vi "RSZVB Marker Bandfilter Results ZVR.vi"(8 "error in (no error)":errorcluster {"code" format="%.0x"}, 9 "Marker (1)":i32=1, 10 "Channel (Trace) (1)":i32=1, 11 "VISA session":refnum<visa-resource-name>) -> (0 "error out":errorcluster {"code" format="%.0x"}, 1 "Bandwidth":dbl format="%^.3e", 3 "dup VISA session":refnum<visa-resource-name>)   [LabVIEW 2011]
doc: "This VI returns the results of a bandpass or a bandstop filter search.\n\nNote(s):\n\n(1) This VI is ZVR compatible.\n\nRemote-control command(s):\nCALCulate<Ch/Tr>:MARKer<Mk>:FUNCtion:BWIDth?"
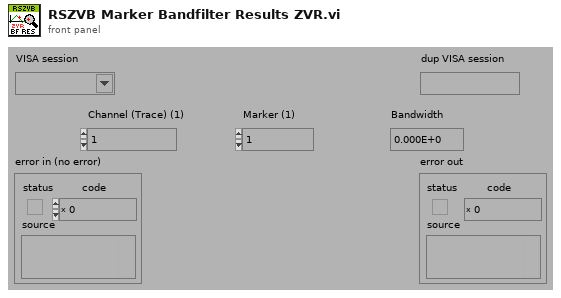
[diagram p1: front panel]
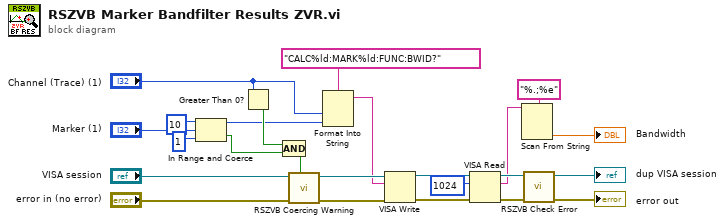
[diagram p0: block diagram]
diagram:
  n1 = In Range and Coerce(upper limit=10, x="Marker (1)", lower limit=1) -> (coerced(x)=w2:i32, In Range?=w12:bool)
  n2 = Greater Than 0?(x="Channel (Trace) (1)") -> (x > 0?=w15:bool)
  n3 = Compound Arithmetic op=AND(w15, w12) -> (w16:bool)
  n4 = call "RSZVB Coercing Warning.vi"("In Range?"=w16, "error in (no error)"="error in (no error)", "VISA session"="VISA session") -> ("error out"=w7:errorcluster, "dup VISA session"=w8:refnum<visa-resource-name>)  [unwired: 7 in]
  n5 = Format Into String(format string="CALC%ld:MARK%ld:FUNC:BWID?", "Channel (Trace) (1)", w2) -> (resulting string=w6:string)  [unwired: 2 in, 1 out]
  n6 = VISA Write(VISA resource name=w8, write buffer=w6, error in (no error)=w7) -> (VISA resource name out=w18:refnum<visa-resource-name>, error out=w19:errorcluster)  [unwired: 1 out]
  n7 = VISA Read(VISA resource name=w18, byte count=u32 1024 ("byte count (0)"), error in (no error)=w19) -> (VISA resource name out=w23:refnum<visa-resource-name>, read buffer=w20:string, error out=w22:errorcluster)  [unwired: 1 out]
  n8 = Scan From String(format string="%.;%e", input string=w20) -> (output 1=→"Bandwidth":dbl)  [unwired: 3 in, 3 out]
  n9 = call "RSZVB Check Error.vi"("error in (no error)"=w22, "VISA session"=w23) -> ("error out"=→"error out":errorcluster, "dup VISA session"=→"dup VISA session":refnum<visa-resource-name>)  [unwired: 8 in]
